vi "Archive files move dir.vi"(5 "hours old date mod(hours)":u8=255, 6 "error in":errorcluster, 7 "File path input cluster":T1={"Archive Location"=path "", "Archive Location 2"=path "<Not A Path>", "OutPut Path"=path "", "Directory(s) To Scan Files"=[]}, 8 "File Management":T2, 9 "Timing True to archive":bool) -> (0 "error IO":errorcluster)   [LabVIEW 2011]
uses:
  Controls/File Management.ctl
  Controls/File Path directories.ctl
  <vilib>/Utility/sysdir.llb/System Directory Type.ctl
panel:
  # "File Handling Method"
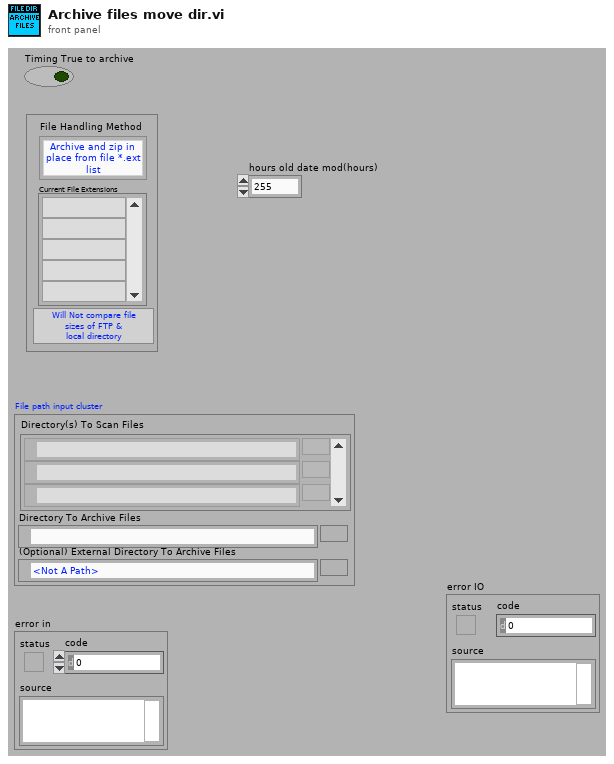
[diagram p1: front panel]
types:
  T1 = typedef "File Path directories.ctl" = cluster{"Archive Location":path, "Archive Location 2":path, "OutPut Path":path, "Directory(s) To Scan Files":path[]}
  T2 = typedef "File Management.ctl" = cluster{"Comp File Size":bool, "File Handle Method":enum16{"Archive and zip in place from file *.ext list", "Archive and zip ALL file Types to archive directory", "Archive and zip to archive directory from file *.ext list", "Perform no file management"}, "file extention list":string[]}
  T3 = enum16{"Archive and zip in place from file *.ext list", "Archive and zip ALL file Types to archive directory", "Archive and zip to archive directory from file *.ext list", "Perform no file management"}
  T4 = typedef "System Directory Type.ctl" = i32
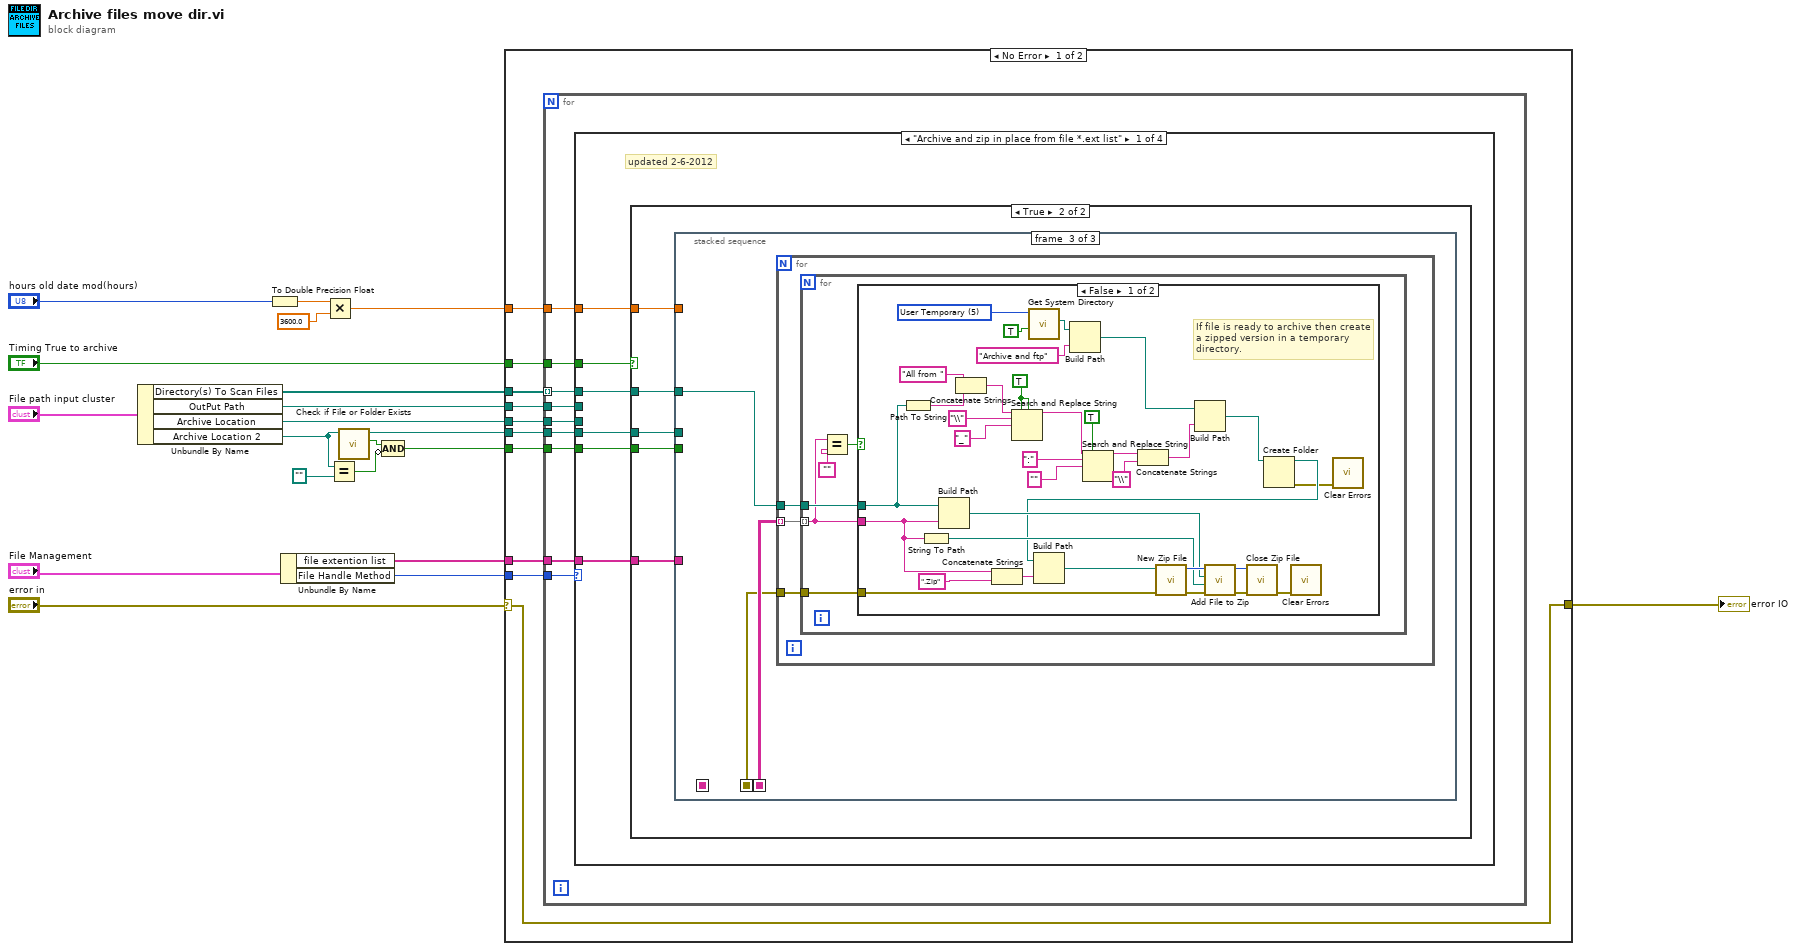
[diagram p0: block diagram]
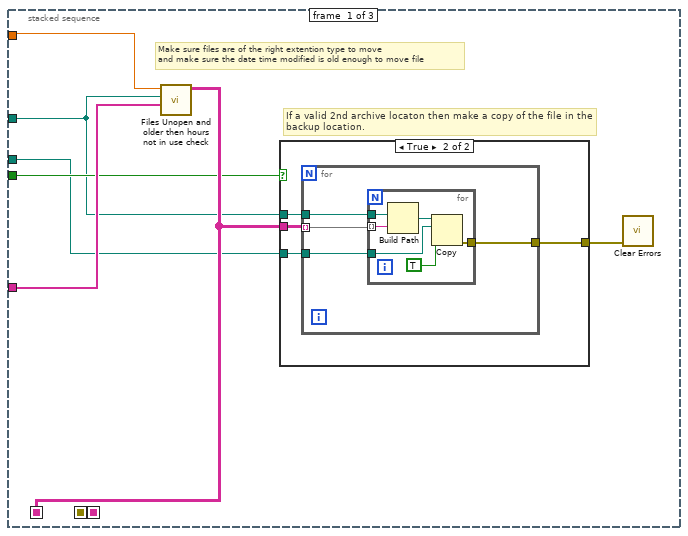
[diagram p3: hidden frame]
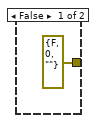
[diagram p4: hidden frame]
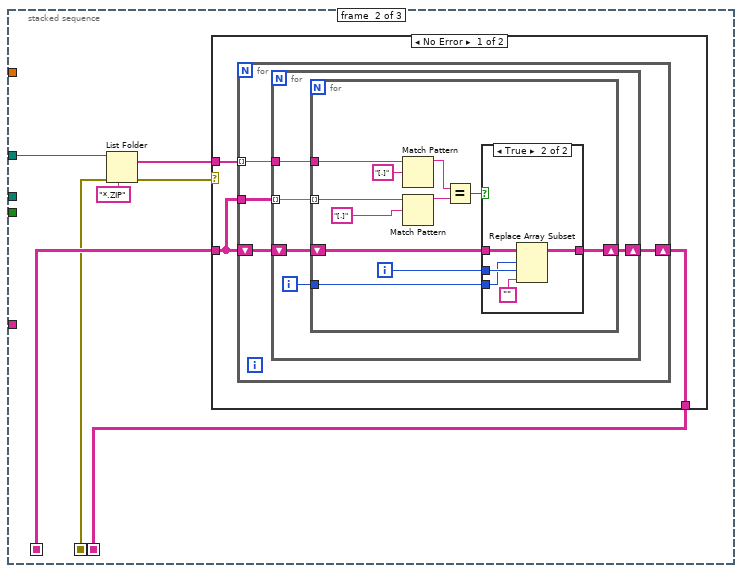
[diagram p5: hidden frame]
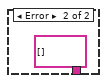
[diagram p7: hidden frame]
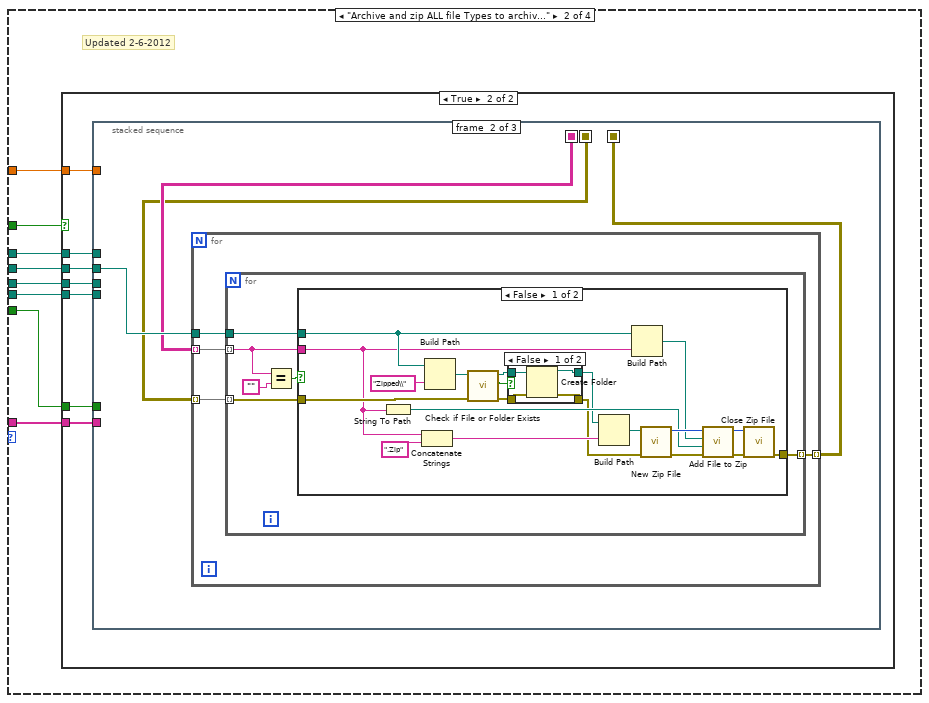
[diagram p9: hidden frame]
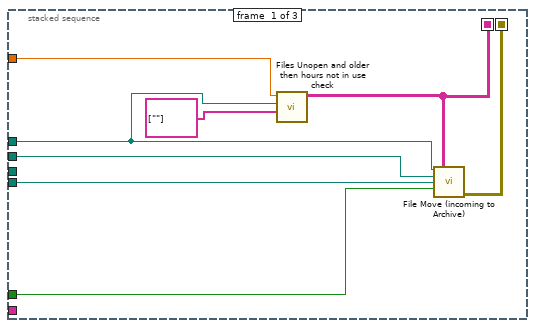
[diagram p11: hidden frame]
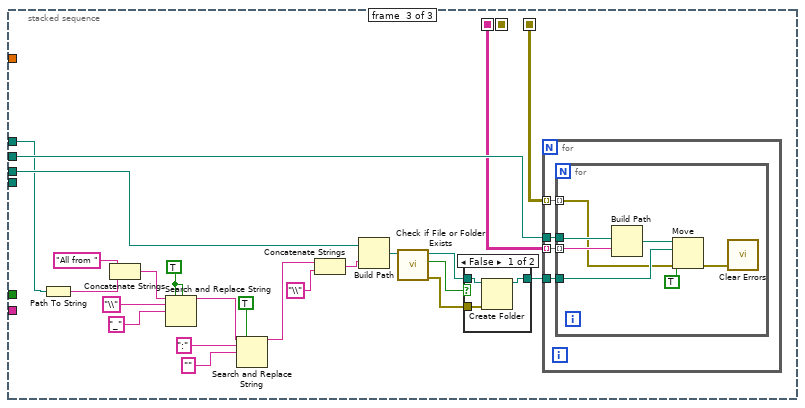
[diagram p14: hidden frame]
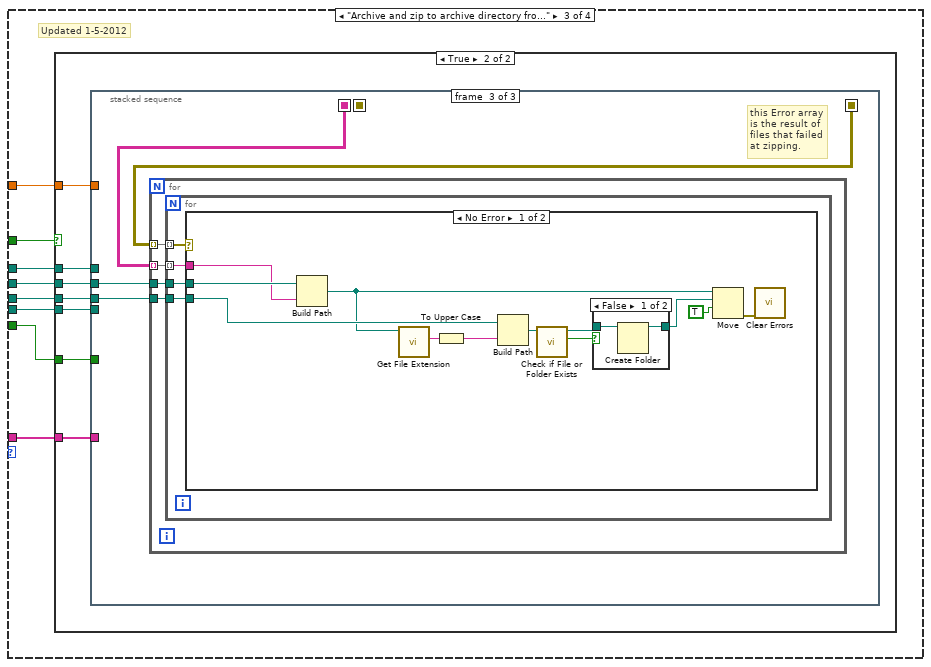
[diagram p16: hidden frame]
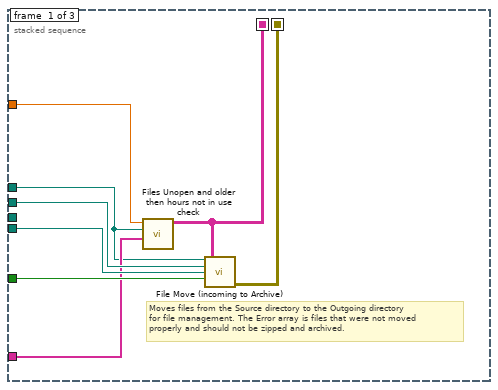
[diagram p18: hidden frame]
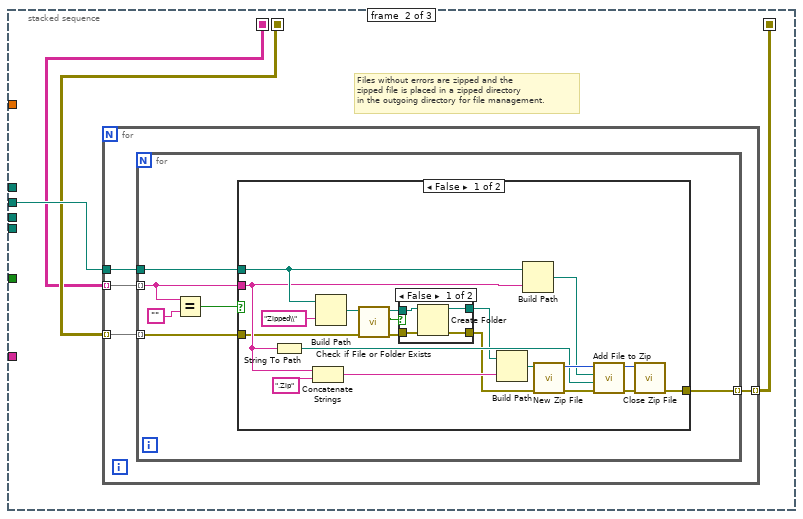
[diagram p19: hidden frame]
diagram:
  n1 = Unbundle By Name("File path input cluster") -> ("Directory(s) To Scan Files"=w10:path[], "OutPut Path"=w9:path, "Archive Location"=w8:path, "Archive Location 2"=w15:path)
  n2 = To Double Precision Float(number="hours old date mod(hours)") -> (double precision float=w3:dbl)
  n3 = Unbundle By Name("File Management") -> ("file extention list"=w16:string[], "File Handle Method"=w18:T3)
  n4 = Multiply(x=w3, y=3600.0) -> (x*y=w4:dbl)
  n5 = Equal?(x=w15, y=path "") -> (x = y?=w12:bool)
  n6 = call <vilib>:"Check if File or Folder Exists.vi"("path"=w15) -> ("file or folder exists?"=w13:bool, "dup path"=w7:path)  [unwired: 8 in, 1 out]
  n7 = Compound Arithmetic op=AND(w13, invert w12) -> (w6:bool)
  n8 = case shown="No Error" "error in" {
    selector: "error in" -> [w21 w347]
    tunnel: "Timing True to archive" -> [w30 _]
    tunnel: [w21 w347] -> w19
    tunnel: w18 -> [w29 _]
    tunnel: w16 -> [w28 _]
    tunnel: w10 -> [w27 _]
    tunnel: w9 -> [w26 _]
    tunnel: w8 -> [w25 _]
    tunnel: w7 -> [w24 _]
    tunnel: w6 -> [w23 _]
    tunnel: w4 -> [w22 _]
    frame No Error {
      n9 = for {
        tunnel: w30 -> [w39]
        tunnel: w29 -> [w38]
        tunnel: w28 -> [w37]
        tunnel: w27 -> [w36] mode=indexing
        tunnel: w26 -> [w35]
        tunnel: w25 -> [w34]
        tunnel: w24 -> [w33]
        tunnel: w23 -> [w32]
        tunnel: w22 -> [w31]
        n10 = case shown="\"Archive and zip in place from file *.ext list\"" w38 {
          tunnel: w39 -> [w45 w161 w263 _]
          tunnel: w36 -> [w44 w160 w262 _]
          tunnel: w35 -> [_ w159 w261 _]
          tunnel: w34 -> [_ w158 w260 _]
          tunnel: w33 -> [w40 w157 w259 _]
          tunnel: w32 -> [w41 w156 w258 _]
          tunnel: w37 -> [w43 w155 w257 _]
          tunnel: w31 -> [w42 w154 w256 _]
          frame "Archive and zip in place from file *.ext list" {
            # "updated 2-6-2012"
            n11 = case shown="True" w45 {
              tunnel: w44 -> [_ w50]
              tunnel: w43 -> [_ w49]
              tunnel: w42 -> [_ w48]
              tunnel: w41 -> [_ w47]
              tunnel: w40 -> [_ w46]
              frame False {
              }
              frame True {
                n12 = stacked-sequence {
                  seq-local: [w55 _ _] -> [_ w75 _]
                  seq-local: [_ w73 _] -> [_ _ w109]
                  seq-local: [_ w74 _] -> [_ _ w111]
                  tunnel: w50 -> [w52 w78 w110]
                  tunnel: w49 -> [w56 _ _]
                  tunnel: w48 -> [w57 _ _]
                  tunnel: w47 -> [w54 _ _]
                  tunnel: w46 -> [w53 _ _]
                  frame #0 {
                    # "If a valid 2nd archive locaton then make a copy of the file in the \nbackup location."
                    # "Make sure files are of the right extention type to move\nand make sure the date time modified is old enough to move file"
                    n13 = call "Files Unopen and older then hours not in use check.vi"("file extention list"=w56, "Dir of Files to move and FTP"=w52, "Time (Hours) last mod must be older then"=w57) -> ("Files to Archive and FTP"=w55:string[][])  [unwired: 8 in]
                    n14 = case shown="True" w54 {
                      tunnel: w55 -> [_ w62]
                      tunnel: w53 -> [_ w61]
                      tunnel: w52 -> [_ w60]
                      tunnel: [errorcluster {"status"=FALSE, "code"=0, "source"=""} ("error out") w59] -> w51
                      frame False {
                      }
                      frame True {
                        n15 = for {
                          tunnel: w61 -> [w66]
                          tunnel: [w63] -> w59
                          tunnel: w60 -> [w65]
                          tunnel: w62 -> [w64] mode=indexing
                          n16 = for {
                            tunnel: w64 -> [w71] mode=indexing
                            tunnel: w65 -> [w72]
                            tunnel: w66 -> [w69]
                            tunnel: [w67] -> w63
                            n17 = Build Path(base path=w72, name or relative path=w71) -> (appended path=w70:path)
                            n18 = Copy(9:TRUE ("overwrite (F)"), 10:w69, 11:w70) -> (0:w67:errorcluster)  [unwired: 2 in, 2 out]
                          }
                        }
                      }
                    }
                    n19 = call <vilib>:"Clear Errors.vi"("error in (no error)"=w51) -> ()  [unwired: 6 in, 1 out]
                  }
                  frame #1 {
                    n20 = List Folder(path=w78, pattern="*.ZIP") -> (filenames=w76:string[], error out=w73:errorcluster)  [unwired: 2 in, 2 out]
                    n21 = case shown="No Error" w73 {
                      tunnel: w76 -> [w81 _]
                      tunnel: w75 -> [w80 _]
                      tunnel: [w79 string[][] [] ("Files to Archive and FTP")] -> w74
                      frame No Error {
                        n22 = for {
                          tunnel: w81 -> [w85] mode=indexing
                          tunnel: w80 -> [w84]
                          shift-right: [w82] -> w79
                          shift-left: w80 -> [w83]
                          n23 = for {
                            tunnel: w85 -> [w89]
                            tunnel: w84 -> [w90] mode=indexing
                            shift-right: [w87] -> w82
                            shift-left: w83 -> [w88]
                            i -> [w86]
                            n24 = for {
                              tunnel: w90 -> [w96] mode=indexing
                              tunnel: w89 -> [w98]
                              tunnel: w86 -> [w93]
                              shift-right: [w95] -> w87
                              shift-left: w88 -> [w92]
                              i -> [w94]
                              n25 = Match Pattern(string=w98, regular expression="[.]") -> (before substring=w97:string)  [unwired: 1 in, 3 out]
                              n26 = Match Pattern(string=w96, regular expression="[.]") -> (before substring=w100:string)  [unwired: 1 in, 3 out]
                              n27 = Equal?(x=w97, y=w100) -> (x = y?=w99:bool)
                              n28 = case shown="True" w99 {
                                tunnel: [w102 w107] -> w95
                                tunnel: w94 -> [_ w104]
                                tunnel: w93 -> [_ w103]
                                tunnel: w92 -> [w102 w105]
                                frame False {
                                }
                                frame True {
                                n29 = Replace Array Subset(array=w105, new element="", index (row)=w103, index (col)=w104) -> (w107:string[][])
                                }
                              }
                            }
                          }
                        }
                      }
                      frame Error {
                      }
                    }
                  }
                  frame #2 {
                    n30 = for {
                      tunnel: w111 -> [w114] mode=indexing
                      tunnel: w110 -> [w113]
                      tunnel: w109 -> [w112]
                      n31 = for {
                        tunnel: w114 -> [w115] mode=indexing
                        tunnel: w113 -> [w118]
                        tunnel: w112 -> [w119]
                        n32 = Equal?(x=w115, y="") -> (x = y?=w117:bool)
                        n33 = case shown="False" w117 {
                          tunnel: w119 -> [w148 _]
                          tunnel: w115 -> [w143 _]
                          tunnel: w118 -> [w126 _]
                          frame False {
                            w131 = TRUE ("replace all? (F)")
                            w139 = T4 5 items=["User Home"=0, "User Desktop"=1, "User Documents"=2, "User Application Data"=3, "User Preferences"=4, "User Temporary"=5, "Public Documents"=6, "Public Application Data"=7, "Public Preferences"=8, "Public Cache"=13, "System Core Libraries"=9, "System Installed Libraries"=10, "Application Files"=11, "Boot Volume Root"=12] ("system directory type")
                            # "If file is ready to archive then create\na zipped version in a temporary\ndirectory."
                            n34 = Path To String(path=w126) -> (string=w135:string)
                            n35 = String To Path(string=w143) -> (path=w149:path)
                            n36 = Build Path(base path=w126, name or relative path=w143) -> (appended path=w144:path)
                            n37 = Concatenate Strings("All from " ("name or relative path"), w135) -> (w134:string)
                            n38 = Concatenate Strings(w143, ".Zip" ("name or relative path")) -> (w145:string)
                            n39 = Search and Replace String(replace all?=w131, case sensitive?=w131, input string=w134, search string="\\" ("replace string (\"\")"), replace string="_" ("replace string (\"\")")) -> (result string=w128:string)  [unwired: 3 in, 3 out]
                            n40 = call <vilib>:"Get System Directory.vi"("create directory if not found? (F)"=TRUE, "system directory type"=w139) -> ("system directory"=w141:path)  [unwired: 9 in]
                            n41 = Build Path(base path=w141, name or relative path="Archive and ftp") -> (appended path=w125:path)
                            n42 = Search and Replace String(replace all?=TRUE ("replace all? (F)"), input string=w128, search string=":" ("replace string (\"\")"), replace string="" ("replace string (\"\")")) -> (result string=w124:string)  [unwired: 4 in, 3 out]
                            n43 = Concatenate Strings(w124, "\\" ("replace string (\"\")")) -> (w122:string)
                            n44 = Build Path(base path=w125, name or relative path=w122) -> (appended path=w121:path)
                            n45 = Create Folder(path (use dialog)=w121) -> (created path=w138:path, error out=w137:errorcluster)  [unwired: 2 in, 1 out]
                            n46 = Build Path(base path=w138, name or relative path=w145) -> (appended path=w147:path)
                            n47 = call <vilib>:"New Zip File.vi"("error in (no error)"=w148, "target"=w147) -> ("error out"=w150:errorcluster, "zip file out"=w153:i64)  [unwired: 3 in, 1 out]
                            n48 = call <vilib>:"Add File to Zip.vi"("error in (no error)"=w150, "destination path in zip"=w149, "source file path"=w144, "zip file in"=w153) -> ("error out"=w152:errorcluster, "zip file out"=w151:i64)  [unwired: 6 in]
                            n49 = call <vilib>:"Close Zip File.vi"("error in (no error)"=w152, "zip file in"=w151) -> ("error out"=w120:errorcluster)  [unwired: 5 in]
                            n50 = call <vilib>:"Clear Errors.vi"("error in (no error)"=w120) -> ()  [unwired: 6 in, 1 out]
                            n51 = call <vilib>:"Clear Errors.vi"("error in (no error)"=w137) -> ()  [unwired: 6 in, 1 out]
                          }
                          frame True {
                          }
                        }
                      }
                    }
                  }
                }
              }
            }
          }
          frame "Archive and zip ALL file Types to archive directory" {
            # "Updated 2-6-2012"
            n52 = case shown="True" w161 {
              tunnel: w160 -> [_ w168]
              tunnel: w158 -> [_ w167]
              tunnel: w157 -> [_ w166]
              tunnel: w156 -> [_ w165]
              tunnel: w159 -> [_ w164]
              tunnel: w155 -> [_ w163]
              tunnel: w154 -> [_ w162]
              frame False {
              }
              frame True {
                n53 = stacked-sequence {
                  seq-local: [w169 _ _] -> [_ w178 w218]
                  seq-local: [w170 _ _] -> [_ w177 _]
                  seq-local: [_ w180 _] -> [_ _ w219]
                  tunnel: w168 -> [w172 _ w228]
                  tunnel: w167 -> [_ _ w237]
                  tunnel: w166 -> [w173 _ _]
                  tunnel: w165 -> [w174 _ _]
                  tunnel: w164 -> [w171 w179 w235]
                  tunnel: w163 -> [_ _ _]
                  tunnel: w162 -> [w175 _ _]
                  frame #0 {
                    n54 = call "Files Unopen and older then hours not in use check.vi"("file extention list"=string[] [""], "Dir of Files to move and FTP"=w172, "Time (Hours) last mod must be older then"=w175) -> ("Files to Archive and FTP"=w169:string[][])  [unwired: 8 in]
                    n55 = call "File Move (incoming to Archive).vi"("source location of files"=w172, "Files to Archive and FTP IN"=w169, "outgoing directory"=w171, "redundant archive location"=w173, "Archive 2 valid path"=w174) -> ("Array of errors from file copy and or move"=w170:errorcluster[][])  [unwired: 10 in]
                  }
                  frame #1 {
                    n56 = for {
                      tunnel: [w184] -> w180 mode=indexing
                      tunnel: w179 -> [w183]
                      tunnel: w178 -> [w182] mode=indexing
                      tunnel: w177 -> [w181] mode=indexing
                      n57 = for {
                        tunnel: w183 -> [w189]
                        tunnel: [w190] -> w184 mode=indexing
                        tunnel: w182 -> [w186] mode=indexing
                        tunnel: w181 -> [w188] mode=indexing
                        n58 = Equal?(x=w186, y="") -> (x = y?=w187:bool)
                        n59 = case shown="False" w187 {
                          tunnel: [w205 w217] -> w190
                          tunnel: w189 -> [w200 _]
                          tunnel: w188 -> [w192 w217]
                          tunnel: w186 -> [w191 _]
                          frame False {
                            n60 = String To Path(string=w191) -> (path=w206:path)
                            n61 = Concatenate Strings(w191, ".Zip" ("name or relative path")) -> (w202:string)
                            n62 = Build Path(base path=w200, name or relative path="Zipped\\") -> (appended path=w198:path)
                            n63 = call <vilib>:"Check if File or Folder Exists.vi"("error in (no error)"=w192, "path"=w198) -> ("error out"=w194:errorcluster, "file or folder exists?"=w197:bool, "dup path"=w196:path)  [unwired: 7 in]
                            n64 = case shown="False" w197 {
                              tunnel: w196 -> [w214 w216]
                              tunnel: [w213 w216] -> w195
                              tunnel: w194 -> [w212 w215]
                              tunnel: [w211 w215] -> w193
                              frame False {
                                n65 = Create Folder(path (use dialog)=w214, error in=w212) -> (created path=w213:path, error out=w211:errorcluster)  [unwired: 1 in, 1 out]
                              }
                              frame True {
                              }
                            }
                            n66 = Build Path(base path=w195, name or relative path=w202) -> (appended path=w204:path)
                            n67 = Build Path(base path=w200, name or relative path=w191) -> (appended path=w201:path)
                            n68 = call <vilib>:"New Zip File.vi"("error in (no error)"=w193, "target"=w204) -> ("error out"=w207:errorcluster, "zip file out"=w210:i64)  [unwired: 3 in, 1 out]
                            n69 = call <vilib>:"Add File to Zip.vi"("error in (no error)"=w207, "destination path in zip"=w206, "source file path"=w201, "zip file in"=w210) -> ("error out"=w209:errorcluster, "zip file out"=w208:i64)  [unwired: 6 in]
                            n70 = call <vilib>:"Close Zip File.vi"("error in (no error)"=w209, "zip file in"=w208) -> ("error out"=w205:errorcluster)  [unwired: 5 in]
                          }
                          frame True {
                          }
                        }
                      }
                    }
                  }
                  frame #2 {
                    w226 = TRUE ("replace all? (F)")
                    n71 = Path To String(path=w228) -> (string=w233:string)
                    n72 = Concatenate Strings("All from " ("name or relative path"), w233) -> (w232:string)
                    n73 = Search and Replace String(replace all?=w226, case sensitive?=w226, input string=w232, search string="\\" ("replace string (\"\")"), replace string="_" ("replace string (\"\")")) -> (result string=w222:string)  [unwired: 3 in, 3 out]
                    n74 = Search and Replace String(replace all?=TRUE ("replace all? (F)"), input string=w222, search string=":" ("replace string (\"\")"), replace string="" ("replace string (\"\")")) -> (result string=w221:string)  [unwired: 4 in, 3 out]
                    n75 = Concatenate Strings(w221, "\\" ("replace string (\"\")")) -> (w225:string)
                    n76 = Build Path(base path=w237, name or relative path=w225) -> (appended path=w240:path)
                    n77 = call <vilib>:"Check if File or Folder Exists.vi"("path"=w240) -> ("error out"=w229:errorcluster, "file or folder exists?"=w239:bool, "dup path"=w238:path)  [unwired: 8 in]
                    n78 = case shown="False" w239 {
                      tunnel: w238 -> [w254 w255]
                      tunnel: [w253 w255] -> w236
                      tunnel: w229 -> [w252 _]
                      frame False {
                        n79 = Create Folder(path (use dialog)=w254, error in=w252) -> (created path=w253:path)  [unwired: 1 in, 2 out]
                      }
                      frame True {
                      }
                    }
                    n80 = for {
                      tunnel: w236 -> [w244]
                      tunnel: w235 -> [w243]
                      tunnel: w219 -> [w242] mode=indexing
                      tunnel: w218 -> [w241] mode=indexing
                      n81 = for {
                        tunnel: w244 -> [w251]
                        tunnel: w243 -> [w247]
                        tunnel: w242 -> [w245] mode=indexing
                        tunnel: w241 -> [w246] mode=indexing
                        n82 = Build Path(base path=w247, name or relative path=w246) -> (appended path=w249:path)
                        n83 = Move(source path=w249, error in=w245, 9:TRUE ("overwrite (F)"), 10:w251) -> (error out=w250:errorcluster)  [unwired: 1 in, 2 out]
                        n84 = call <vilib>:"Clear Errors.vi"("error in (no error)"=w250) -> ()  [unwired: 6 in, 1 out]
                      }
                    }
                  }
                }
              }
            }
          }
          frame "Archive and zip to archive directory from file *.ext list" {
            # "Updated 1-5-2012"
            n85 = case shown="True" w263 {
              tunnel: w262 -> [_ w270]
              tunnel: w260 -> [_ w269]
              tunnel: w259 -> [_ w268]
              tunnel: w258 -> [_ w267]
              tunnel: w261 -> [_ w266]
              tunnel: w257 -> [_ w265]
              tunnel: w256 -> [_ w264]
              frame False {
              }
              frame True {
                n86 = stacked-sequence {
                  seq-local: [w273 _ _] -> [_ w280 w320]
                  seq-local: [w274 _ _] -> [_ w281 _]
                  seq-local: [_ w279 _] -> [_ _ w321]
                  tunnel: w270 -> [w271 _ _]
                  tunnel: w269 -> [_ _ w323]
                  tunnel: w268 -> [w277 _ _]
                  tunnel: w267 -> [w278 _ _]
                  tunnel: w266 -> [w276 w282 w322]
                  tunnel: w265 -> [w272 _ _]
                  tunnel: w264 -> [w275 _ _]
                  frame #0 {
                    # "Moves files from the Source directory to the Outgoing directory\nfor file management. The Error array is files that were not moved\nproperly and should not be zipped and archived."
                    n87 = call "Files Unopen and older then hours not in use check.vi"("file extention list"=w272, "Dir of Files to move and FTP"=w271, "Time (Hours) last mod must be older then"=w275) -> ("Files to Archive and FTP"=w273:string[][])  [unwired: 8 in]
                    n88 = call "File Move (incoming to Archive).vi"("source location of files"=w271, "Files to Archive and FTP IN"=w273, "outgoing directory"=w276, "redundant archive location"=w277, "Archive 2 valid path"=w278) -> ("Array of errors from file copy and or move"=w274:errorcluster[][])  [unwired: 10 in]
                  }
                  frame #1 {
                    # "Files without errors are zipped and the \nzipped file is placed in a zipped directory\nin the outgoing directory for file management."
                    n89 = for {
                      tunnel: w282 -> [w286]
                      tunnel: w280 -> [w285] mode=indexing
                      tunnel: w281 -> [w284] mode=indexing
                      tunnel: [w283] -> w279 mode=indexing
                      n90 = for {
                        tunnel: w286 -> [w292]
                        tunnel: w285 -> [w290] mode=indexing
                        tunnel: w284 -> [w287] mode=indexing
                        tunnel: [w288] -> w283 mode=indexing
                        n91 = Equal?(x=w290, y="") -> (x = y?=w291:bool)
                        n92 = case shown="False" w291 {
                          tunnel: w292 -> [w303 _]
                          tunnel: w290 -> [w295 _]
                          tunnel: [w294 errorcluster {"status"=TRUE, "code"=0, "source"=""} ("error out")] -> w288
                          tunnel: w287 -> [w293 _]
                          frame False {
                            n93 = String To Path(string=w295) -> (path=w308:path)
                            n94 = Concatenate Strings(w295, ".Zip" ("name or relative path")) -> (w305:string)
                            n95 = Build Path(base path=w303, name or relative path="Zipped\\") -> (appended path=w301:path)
                            n96 = call <vilib>:"Check if File or Folder Exists.vi"("error in (no error)"=w293, "path"=w301) -> ("error out"=w297:errorcluster, "file or folder exists?"=w300:bool, "dup path"=w299:path)  [unwired: 7 in]
                            n97 = case shown="False" w300 {
                              tunnel: w299 -> [w316 w318]
                              tunnel: [w315 w318] -> w298
                              tunnel: w297 -> [w314 w317]
                              tunnel: [w313 w317] -> w296
                              frame False {
                                n98 = Create Folder(path (use dialog)=w316, error in=w314) -> (created path=w315:path, error out=w313:errorcluster)  [unwired: 1 in, 1 out]
                              }
                              frame True {
                              }
                            }
                            n99 = Build Path(base path=w298, name or relative path=w305) -> (appended path=w307:path)
                            n100 = Build Path(base path=w303, name or relative path=w295) -> (appended path=w304:path)
                            n101 = call <vilib>:"New Zip File.vi"("error in (no error)"=w296, "target"=w307) -> ("error out"=w309:errorcluster, "zip file out"=w312:i64)  [unwired: 3 in, 1 out]
                            n102 = call <vilib>:"Add File to Zip.vi"("error in (no error)"=w309, "destination path in zip"=w308, "source file path"=w304, "zip file in"=w312) -> ("error out"=w311:errorcluster, "zip file out"=w310:i64)  [unwired: 6 in]
                            n103 = call <vilib>:"Close Zip File.vi"("error in (no error)"=w311, "zip file in"=w310) -> ("error out"=w294:errorcluster)  [unwired: 5 in]
                          }
                          frame True {
                          }
                        }
                      }
                    }
                  }
                  frame #2 {
                    # "this Error array \nis the result of \nfiles that failed\nat zipping."
                    n104 = for {
                      tunnel: w323 -> [w327]
                      tunnel: w322 -> [w326]
                      tunnel: w321 -> [w325] mode=indexing
                      tunnel: w320 -> [w324] mode=indexing
                      n105 = for {
                        tunnel: w327 -> [w331]
                        tunnel: w326 -> [w330]
                        tunnel: w325 -> [w329] mode=indexing
                        tunnel: w324 -> [w328] mode=indexing
                        n106 = case shown="No Error" w329 {
                          tunnel: w331 -> [w343 _]
                          tunnel: w330 -> [w337 _]
                          tunnel: w328 -> [w335 _]
                          frame No Error {
                            n107 = Build Path(base path=w337, name or relative path=w335) -> (appended path=w334:path)
                            n108 = call <vilib>:"Get File Extension.vi"("file"=w334) -> ("lowercase file extension"=w333:string)  [unwired: 7 in, 3 out]
                            n109 = To Upper Case(1:w333) -> (0:w332:string)
                            n110 = Build Path(base path=w343, name or relative path=w332) -> (appended path=w342:path)
                            n111 = call <vilib>:"Check if File or Folder Exists.vi"("path"=w342) -> ("file or folder exists?"=w341:bool, "dup path"=w340:path)  [unwired: 8 in, 1 out]
                            n112 = case shown="False" w341 {
                              tunnel: w340 -> [w345 w346]
                              tunnel: [w344 w346] -> w339
                              frame False {
                                n113 = Create Folder(path (use dialog)=w345) -> (created path=w344:path)  [unwired: 2 in, 2 out]
                              }
                              frame True {
                              }
                            }
                            n114 = Move(source path=w334, 9:TRUE ("overwrite (F)"), 10:w339) -> (error out=w336:errorcluster)  [unwired: 2 in, 2 out]
                            n115 = call <vilib>:"Clear Errors.vi"("error in (no error)"=w336) -> ()  [unwired: 6 in, 1 out]
                          }
                          frame Error {
                          }
                        }
                      }
                    }
                  }
                }
              }
            }
          }
          frame "Perform no file management", Default {
          }
        }
      }
    }
    frame Error {
    }
  }
  "error IO" <- w19
